vi "test_fpga_resources.vi"() -> ()   [LabVIEW 2017]
uses:
  <vilib>/NI/LVFPGA Adv Session Resources/LVFPGAAdvSessionResources.lvlib
  <vilib>/NI/LVFPGA Adv Session Resources/OpenByName.xnode
  <vilib>/rvi/interface/nirviCloseFPGA/nirviCloseFPGA.xnode
  <vilib>/FPGAPlugInAG/Dynamic/niLvFpga_Close_Dynamic.vi
  <vilib>/NI/LVFPGA Adv Session Resources/OpenByName (SubVI).vi
  <vilib>/rvi/interface/nirviReadWriteControl/nirviReadWriteControl.xnode
  NiFpgaLv.dll
  <vilib>/Utility/error.llb/Error Cluster From Error Code.vi
  <vilib>/rvi/interface/Simulation/niFpgaSimulationCallBeginRW.vi
  <vilib>/rvi/errors/niLvFpgaAdjustHostInterfaceError.vi
  <vilib>/NI/LVFPGA Adv Session Resources/OpenByNameSubVI.vi
  <vilib>/rvi/interface/nirviMethod/nirviMethod.xnode
  <vilib>/FPGAPlugInAG/Dynamic/niLvFpga_P2PGetEndpoint_Dynamic.vi
  <vilib>/rvi/errors/niLvFpgaMergeErrorWithErrorCode.vi
  <vilib>/NI/LVFPGA Adv Session Resources/ResourceInfo.ctl
  Program Files (x86)/National Instruments/LabVIEW 2013/examples/NI/LVFPGA Adv Session Resources/Knock Sensor Interface.ctl
panel:
  out "error out":errorcluster
  in  "KnockSensor.Mine":T1
  in  "Bitfile path 2":path
  out "First resource type":T2(ring)
  out "First data type":variant
  out "First resource name":string
  in  "Device address":string="PXI1Slot3"
  out "Resource info out":T3[](array[typedef])=[{"Resource name"="Data Read", "Data type"=variant(u64 0), "Resource type"=enum."Register"}, {"Resource name"="Data Valid?", "Data type"=variant(bool FALSE), "Resource type"=enum."Register"}, {"Resource name"="Data Expected", "Data type"=variant(u64 0), "Resource type"=enum."Register"}, {"Resource name"="p2p reader", "Data type"=variant(u64 0), "Resource type"=enum."Host To Target FIFO"}]
  in  "Bitfile path":path=path "C:/Program Files (x86)/National Instruments/LabVIEW 2017/examples/R Series/Device Specific/PXIe DIO Devices/Peer to Peer Streaming/FPGA Bitfiles/PeertoPeerStream_FPGATarget2_PeerToPeerReader_ZvmxKEr8-yg.lvbitx"
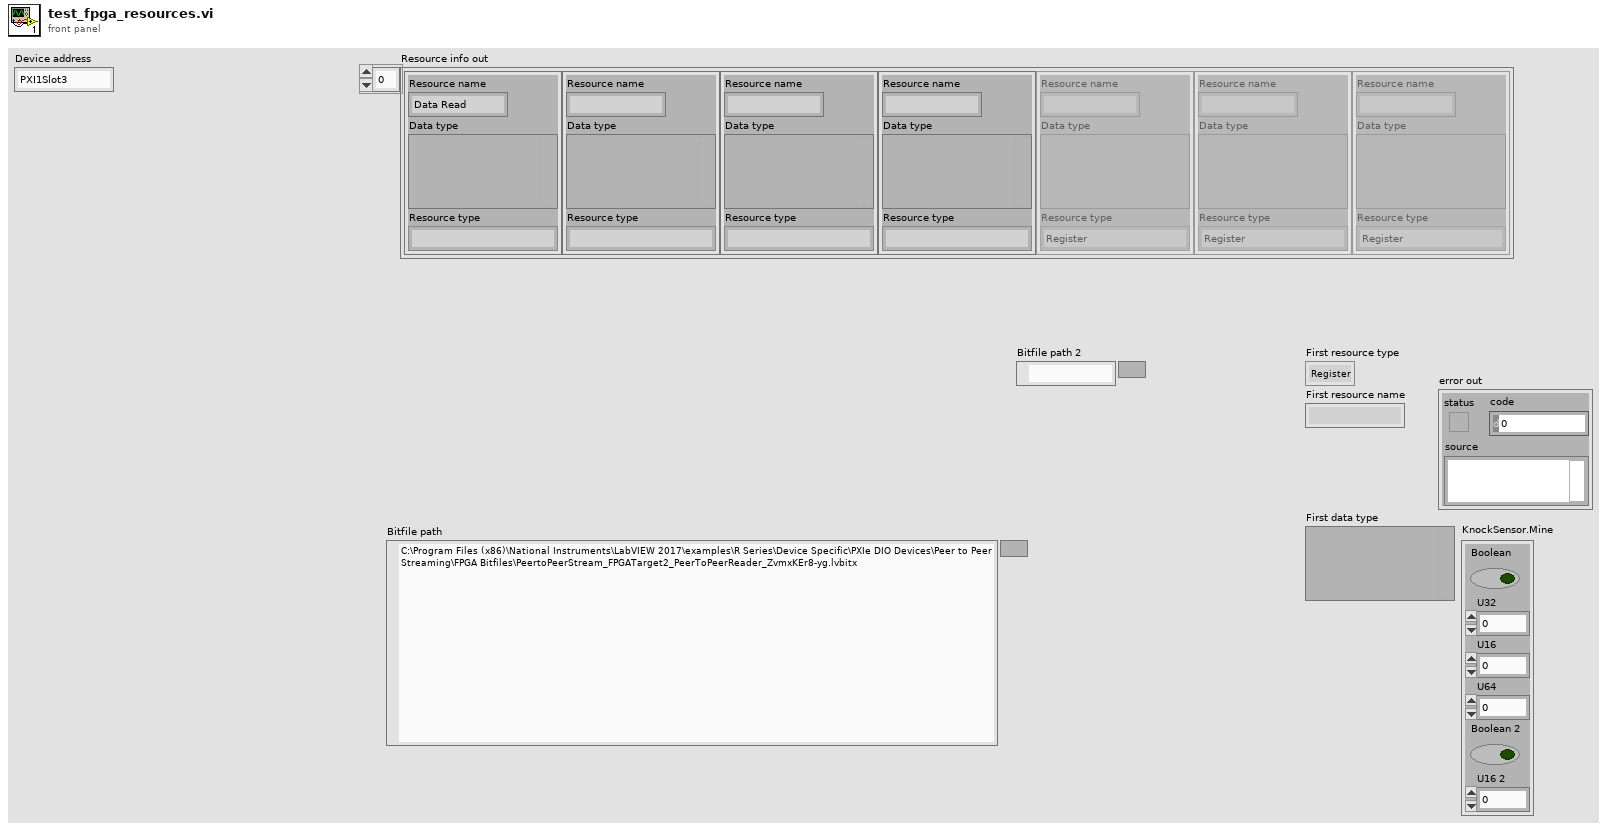
[diagram p1: front panel]
types:
  T1 = typedef "Knock Sensor Interface.ctl" = cluster{"Boolean":bool, "U32":u32, "U16":u16, "U64":u64, "Boolean 2":bool, "U16 2":u16}
  T2 = enum16{"Register", "Host To Target FIFO", "Target To Host FIFO"}
  T3 = typedef "LVFPGAAdvSessionResources.lvlib/ResourceInfo.ctl" = cluster{"Resource name":string, "Data type":variant, "Resource type":enum16{"Register", "Host To Target FIFO", "Target To Host FIFO"}}
  T4 = typedef "LVFPGA Adv Session Resources.lvlib/ResourceInfo.ctl" = cluster{"Resource name":string, "Data type":variant, "Resource type":enum16{"Register", "Host To Target FIFO", "Target To Host FIFO"}}
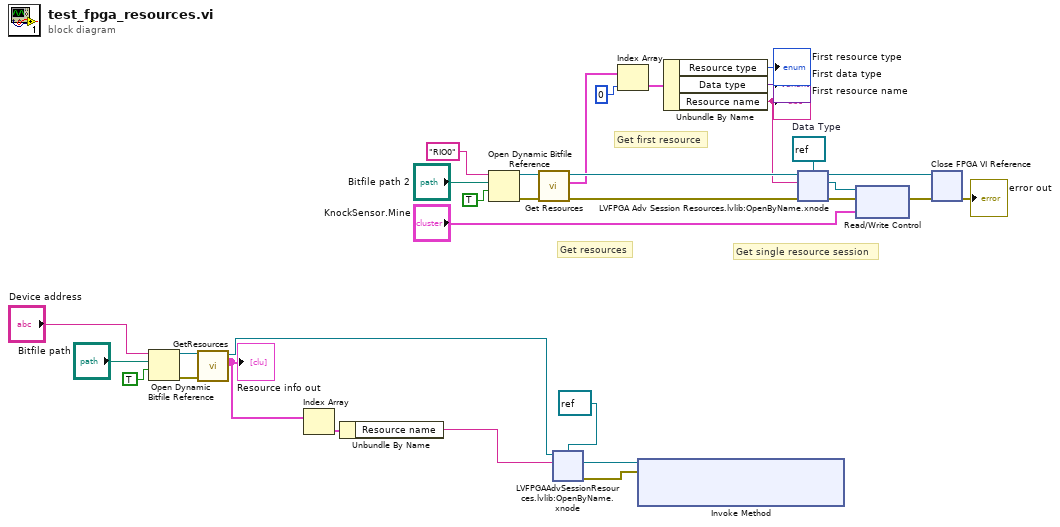
[diagram p0: block diagram]
diagram:
  w14 = refnum<k20> refnum  # Data Type
  # "Get single resource session"
  # "Get resources"
  # "Get first resource"
  n1 = Open Dynamic Bitfile Reference(0:"Device address", 1:"Bitfile path", 2:TRUE ("Run When Loaded")) -> (5:w28:refnum<k20>, 8:w29:errorcluster)  [unwired: 2 in]
  n2 = call <vilib>:"GetResources.vi"("error in (no error)"=w29, "FPGA VI Reference in"=w28) -> ("Resource info out"=w27:T3[], "FPGA VI Reference out"=w24:refnum<k20>)  [unwired: 7 in, 1 out]
  "Resource info out" <- w27
  n3 = Index Array(array=w27) -> (element=w26:T3)  [unwired: 1 in]
  n4 = Unbundle By Name(w26) -> ("Resource name"=w25:string)
  n5 = Open Dynamic Bitfile Reference(0:"RIO0" ("Device address"), 1:"Bitfile path 2", 2:TRUE ("Run When Loaded")) -> (5:w21:refnum<k20>, 8:w22:errorcluster)  [unwired: 2 in]
  n6 = call <vilib>:"Get Resources.vi"("error in (no error)"=w22, "FPGA VI Reference in"=w21) -> ("error out"=w19:errorcluster, "Resource info out"=w10:T4[], "FPGA VI Reference out"=w17:refnum<k20>)  [unwired: 7 in]
  n7 = xnode "LVFPGAAdvSessionResources.lvlib:OpenByName.xnode"("FPGA VI Reference in"=w24, "Resource name in"=w25, "Single resource reference type in"=refnum<k20> refnum ("FPGA Interface")) -> ("Single resource reference out"=w2:refnum<k20>, "Error out"=w1:errorcluster)  [unwired: 1 in, 1 out]
  n8 = Index Array(array=w10, index=0) -> (element=w7:T4)
  n9 = xnode "Invoke Method"("FPGA VI Reference In"=w2, "error in"=w1) -> ()  [unwired: 3 out]
  n10 = Unbundle By Name(w7) -> ("Resource type"=→"First resource type":T2, "Data type"=→"First data type":variant, "Resource name"=w4:string)
  "First resource name" <- w4
  n11 = xnode "LVFPGA Adv Session Resources.lvlib:OpenByName.xnode"("FPGA VI Reference in"=w17, "Resource name in"=w4, "Single resource reference type in"=w14, "Error in"=w19) -> ("Single resource reference out"=w12:refnum<k20>, "Error out"=w15:errorcluster, "FPGA VI Reference out"=w18:refnum<k20>)
  n12 = xnode "Read/Write Control"("FPGA VI Reference In"=w12, "error in"=w15, "Value"="KnockSensor.Mine") -> ("error out"=w13:errorcluster)  [unwired: 1 out]
  n13 = xnode "Close FPGA VI Reference"("FPGA VI Reference In"=w18, "error in"=w13) -> ("error out"=→"error out":errorcluster)
